vi "rotina de aquisição dos dados de calibracao.vi"() -> ()   [LabVIEW 2011]
uses:
  <vilib>/express/express analysis/Spectral/XNode/ExpressSpectralMeasurementsBlockNode.xnode
  <vilib>/express/express analysis/Spectral/Block/exnSpectralBlock spectral measurements power poly.vi
  <vilib>/express/express analysis/Spectral/Block/exnSpectralBlock spectral measurements power DDT.vi
  <vilib>/express/express analysis/Spectral/Block/exnSpectralBlock spectral measurements power WFM.vi
  <vilib>/Analysis/NI_AALPro.lvlib
  <vilib>/Analysis/polynomials.llb/1D Polynomial Evaluation (DBL).vi
panel:
  out "calibracao":dbl[](array[numeric])
  out "Power Spectrum":cluster{"f0":dbl, "df":dbl, "magnitude":dbl[]}(graph)
  in  "Upper Cut-Off":dbl=65.0
  out "Waveform Graph":dynamicdata(graph)
  in  "Frequência de Corte (Hz)":dbl=60.0 caption="Lower Cut-Off"
  out "Gráfico - tempo real/sinal bruto":dbl[](graph) caption="Gráfico - tempo real/bruto"
  in  "stop":bool
  out "Gráfico - tempo real/sinal filtrado":dbl[](graph) caption="Gráfico - tempo real/filtrado"
  out "Gráfico 2":waveform(dbl)(graph)
  in  "Parar programa":bool
  in  "OK Button":bool
  out "direito":dbl
  out "esquerdo":dbl
  # "PROGRAMA DE AQUISIÇÃO DE SINAL PARA CARACTERIZAÇÃO"
  # "SINAL AQUISITADO EM TEMPO REAL"
  # "SINAL A SER GRAVADO PARA PROCESSAMENTO"
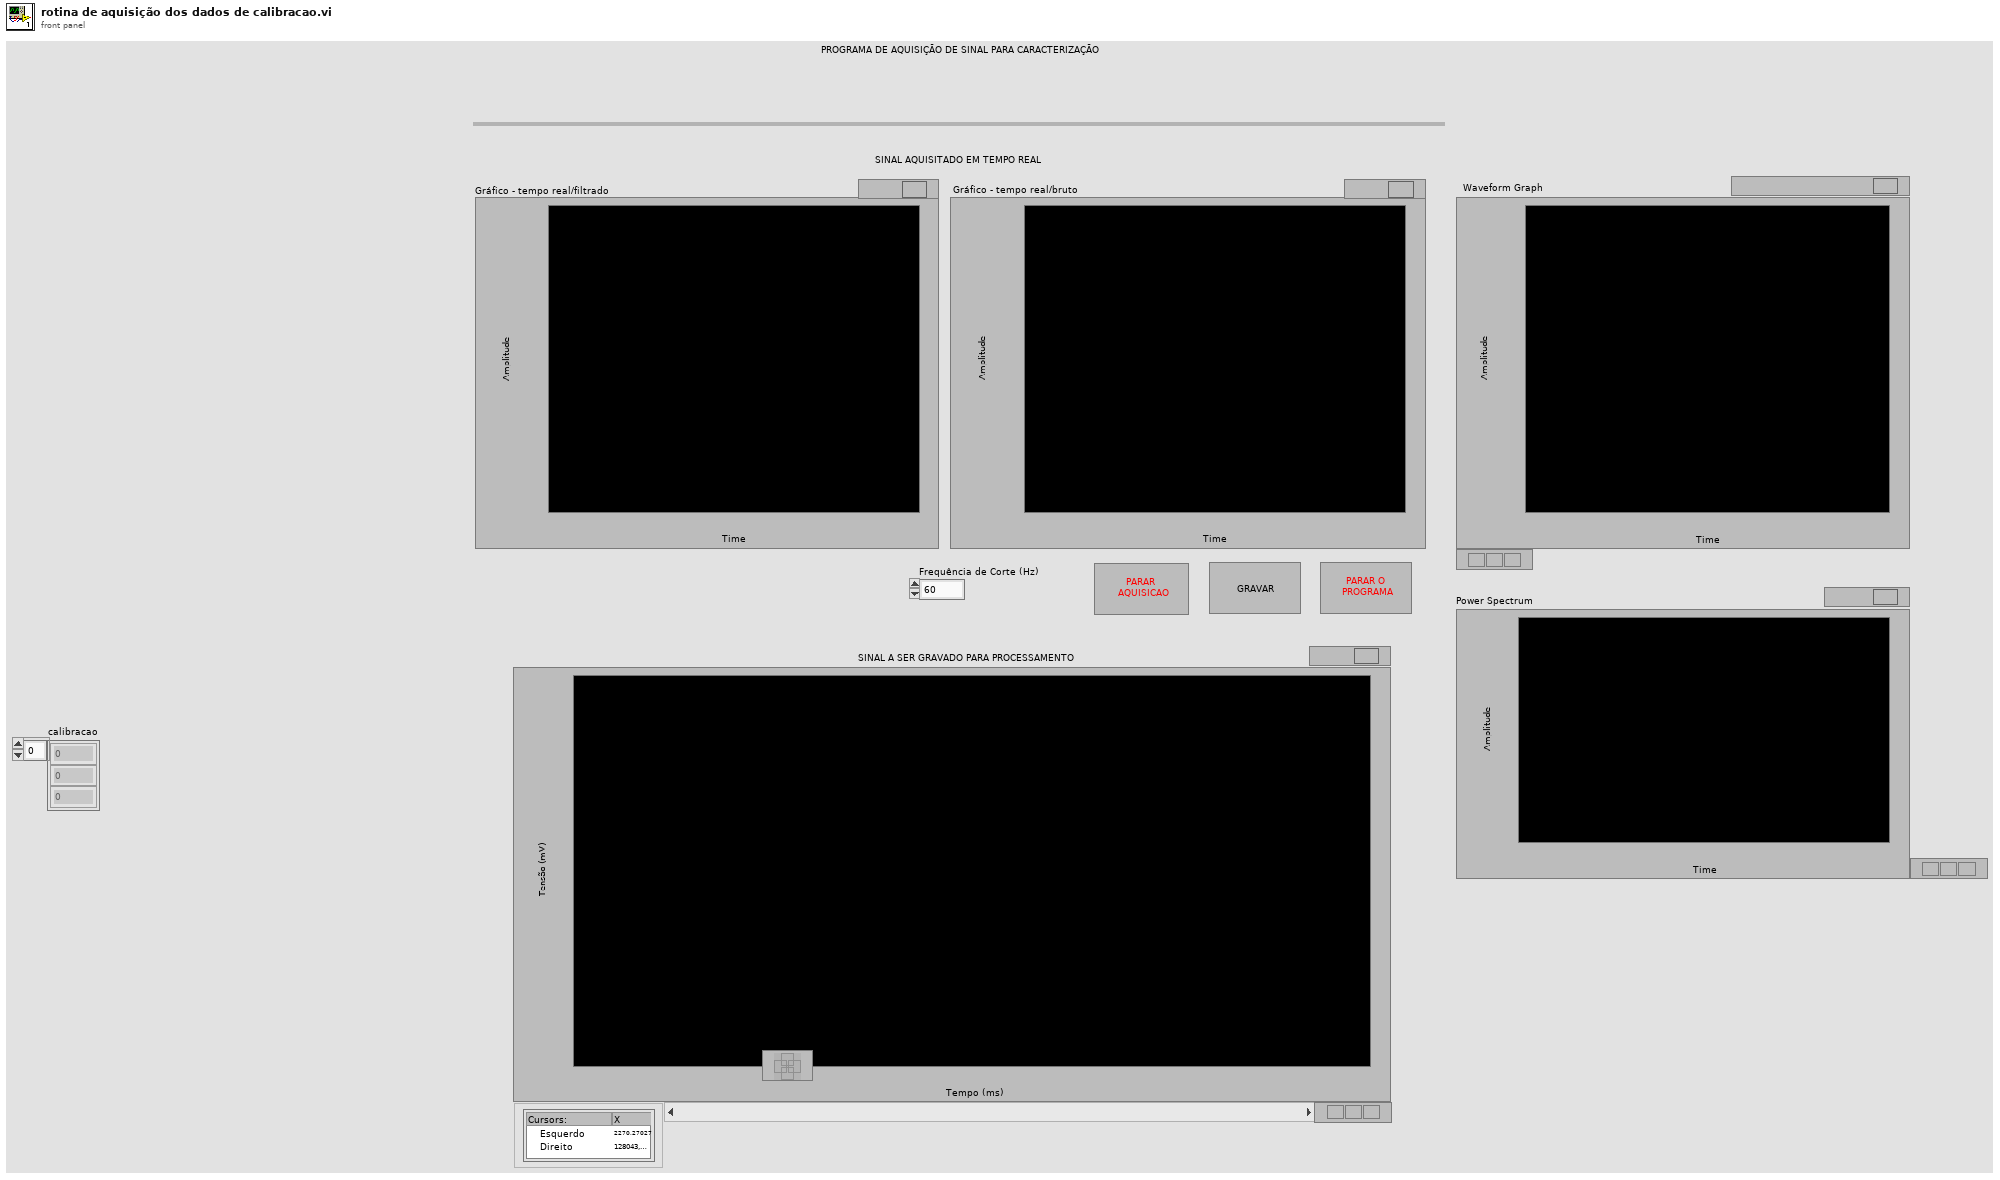
[diagram p1: front panel]
types:
  T1 = cluster{"averaging mode":u16, "weighting mode":u16, "number of averages":u32}
  T2 = cluster{"dB On (F)":bool, "unwrap phase (F)":bool, "convert to degree (F)":bool}
  T3 = typedef "NI_Matrix.lvlib/RealMatrix.ctl" = dbl[][]
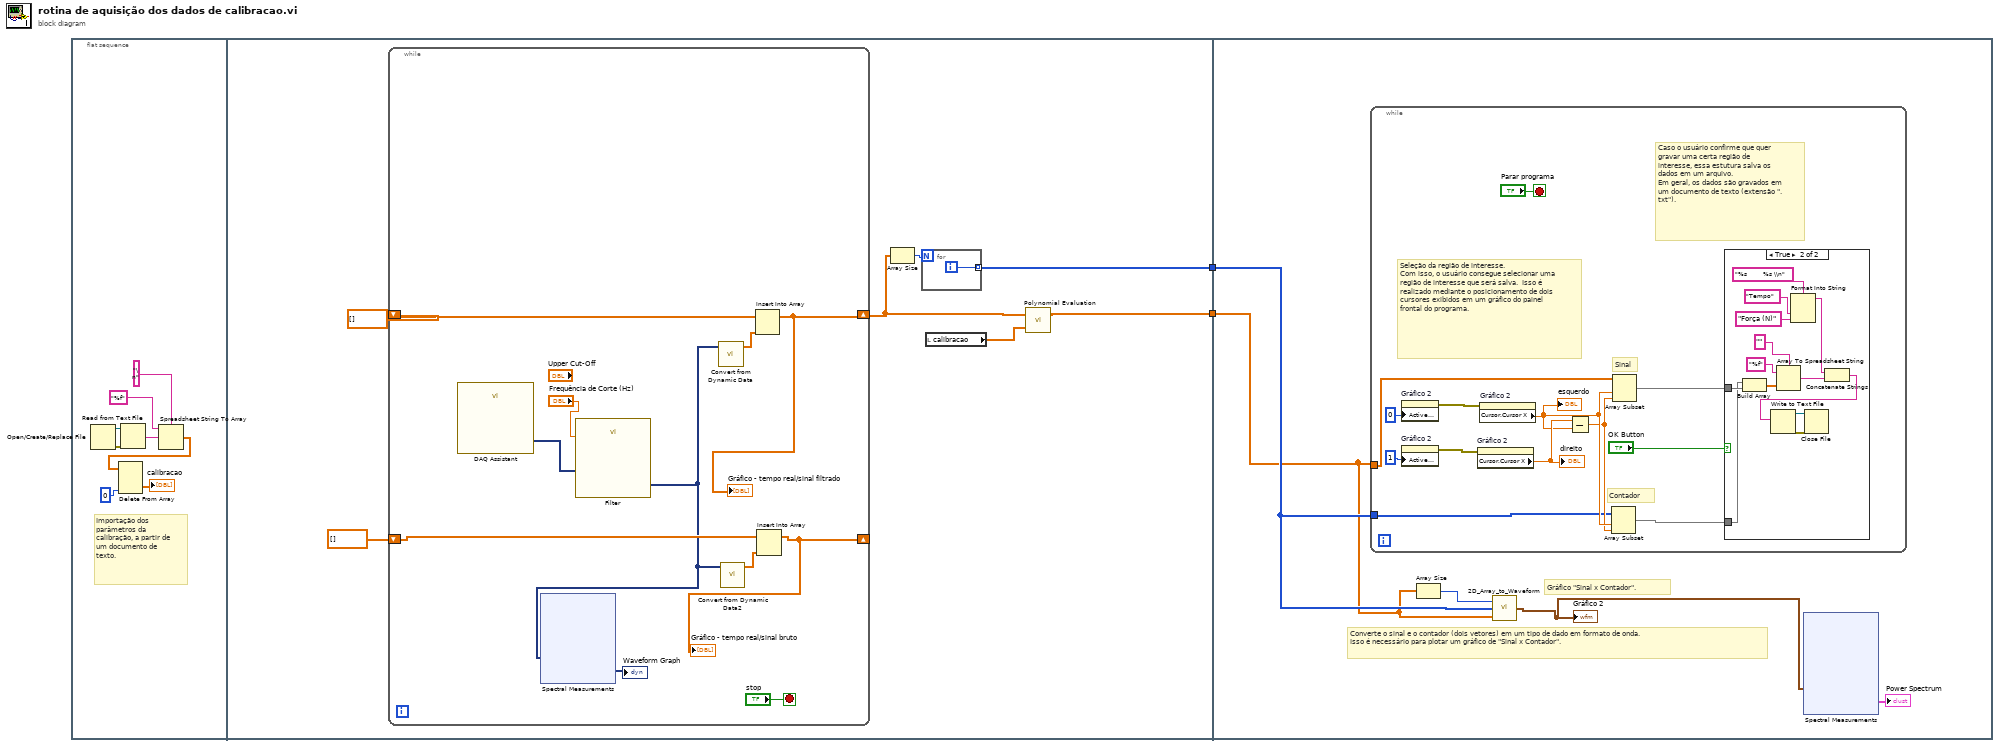
[diagram p0: block diagram]
diagram:
  n1 = flat-sequence {
    tunnel: [w15] -> w2
    tunnel: [w11] -> w1
    tunnel: w2 -> [w42]
    tunnel: w1 -> [w41]
    frame #0 {
      # "Importação dos parâmetros da calibração, a partir de um documento de texto."
      n2 = Open/Create/Replace File() -> (refnum out=w5:refnum<file>, error out=w6:errorcluster)  [unwired: 6 in, 1 out]
      n3 = Read from Text File(file (use dialog)=w5, error in=w6) -> (text=w4:string)  [unwired: 2 in, 3 out]
      n4 = Spreadsheet String To Array(delimiter (Tab)="\n", format string="%f", spreadsheet string=w4) -> (array=w3:dbl[][])  [unwired: 1 in]
      n5 = Delete From Array(array=w3, index (col)=0 ("disabled index (col)")) -> (deleted portion=→"calibracao":dbl[])  [unwired: 2 in, 1 out]
    }
    frame #1 {
      n6 = while {
        shift-right: [w26] -> w12
        shift-left: dbl[] [] ("Array") -> [w28]
        shift-right: [w23] -> _
        shift-left: dbl[] [] ("Array") -> [w24]
        stop <- "stop" stop-if-true
        n7 = call "DAQ Assistant"() -> ("data"=w21:dynamicdata)  [unwired: 16 in, 3 out]
        n8 = call "Filter"("Lower Cut-Off"="Frequência de Corte (Hz)", "Signal"=w21) -> ("Filtered Signal"=w20:dynamicdata)  [unwired: 8 in, 1 out]
        n9 = xnode "Spectral Measurements"("Signals"=w20) -> ("Power Spectrum"=→"Waveform Graph":dynamicdata)  [unwired: 1 in, 1 out]
        n10 = call "Convert from Dynamic Data"("Dynamic Data Type"=w20) -> ("Array"=w29:dbl[])  [unwired: 3 in]
        n11 = call "Convert from Dynamic Data2"("Dynamic Data Type"=w20) -> ("Array"=w25:dbl[])  [unwired: 3 in]
        n12 = Insert Into Array(array=w28, new element=w29) -> (w26:dbl[])  [unwired: 1 in]
        "Gráfico - tempo real/sinal filtrado" <- w26
        n13 = Insert Into Array(array=w24, new element=w25) -> (w23:dbl[])  [unwired: 1 in]
        "Gráfico - tempo real/sinal bruto" <- w23
      }
      n14 = Array Size(array=w12) -> (size(s)=w16:i32)
      n15 = for {
        N: w16 -> [_]
        tunnel: [w18] -> w15 mode=indexing
        i -> [w18]
      }
      n16 = local read "calibracao"() -> (w13:dbl[])
      n17 = call-poly <vilib>:"Polynomial Evaluation.vi"("P(x)"=w13, "A"=w12) -> ("P(A)"=w11:dbl[])  [unwired: 1 out]
    }
    frame #2 {
      # "Gráfico \"Sinal x Contador\"."
      # "Converte o sinal e o contador (dois vetores) em um tipo de dado em formato de onda. \nIsso é necessário para plotar um gráfico de \"Sinal x Contador\"."
      n18 = while {
        tunnel: w42 -> [w55]
        tunnel: w41 -> [w53]
        stop <- "Parar programa" stop-if-true
        # "Caso o usuário confirme que quer gravar uma certa região de interesse, essa estutura salva os dados em um arquivo.\nEm geral, os dados são gravados em um documento de texto (extensão \".txt\")."
        # "Seleção da região de interesse. \nCom isso, o usuário consegue selecionar uma região de interesse que será salva.  Isso é realizado mediante o posicionamento de dois cursores exibidos em um gráfico do painel frontal do programa."
        # "Contador"
        # "Sinal"
        n19 = property on="Gráfico 2" class="WFGraph (strict)"("Active Cursor"=u32 0) -> (error out=w65:errorcluster)  [unwired: 2 in, 1 out]
        n20 = property on="Gráfico 2" class="WFGraph (strict)"("Active Cursor"=u32 1) -> (error out=w63:errorcluster)  [unwired: 2 in, 1 out]
        n21 = property on="Gráfico 2" class="WFGraph (strict)"(error in=w63) -> ("Cursor.Cursor X"=w61:dbl)  [unwired: 1 in, 2 out]
        "direito" <- w61
        n22 = property on="Gráfico 2" class="WFGraph (strict)"(error in=w65) -> ("Cursor.Cursor X"=w57:dbl)  [unwired: 1 in, 2 out]
        "esquerdo" <- w57
        n23 = Subtract(x=w61, y=w57) -> (x-y=w56:dbl)
        n24 = Array Subset(array=w55, index=w57, length=w56) -> (w54:i32[])
        n25 = Array Subset(array=w53, index=w57, length=w56) -> (w59:dbl[])
        n26 = case shown="True" "OK Button" {
          tunnel: w59 -> [_ w67]
          tunnel: w54 -> [_ w66]
          frame False {
          }
          frame True {
            n27 = Build Array(w66, w67) -> (w71:T3)
            n28 = Array To Spreadsheet String(delimiter (Tab)="", array=w71, 3:"%f" ("format string")) -> (spreadsheet string=w73:string)
            n29 = Format Into String(format string="%s        %s \\n", "Tempo" ("input 1"), "Força (N)" ("input 2")) -> (resulting string=w72:string)  [unwired: 2 in, 1 out]
            n30 = Concatenate Strings(w72, w73) -> (w68:string)
            n31 = Write to Text File(text=w68) -> (refnum out=w70:refnum<file>, error out=w69:errorcluster)  [unwired: 3 in, 1 out]
            n32 = Close File(refnum=w70, error in=w69) -> ()  [unwired: 2 out]
          }
        }
      }
      n33 = Array Size(array=w41) -> (size(s)=w43:i32)
      n34 = call "2D_Array_to_Waveform.vi"("Y"=w41, "X"=w42, "Nº de amostras"=w43) -> ("output waveform"=w40:waveform(dbl))
      "Gráfico 2" <- w40
      n35 = xnode "Spectral Measurements"("Signals"=w40) -> ("Power Spectrum"=→"Power Spectrum":cluster{"f0":dbl, "df":dbl, "magnitude":dbl[]})  [unwired: 1 in, 1 out]
    }
  }
